vi "time_frequency.vi"() -> ()   [LabVIEW 2018]
uses:
  <vilib>/addons/Time Frequency Analysis/Spectrogram.llb/TFA Adaptive Spectrogram (Waveform).vi
  <vilib>/addons/Time Frequency Analysis/Spectrogram.llb/TFA Choi-Williams Distribution (Waveform).vi
  <vilib>/addons/Time Frequency Analysis/Transform.llb/TFA STFT (Waveform).vi
  <vilib>/addons/_Advanced Signal Processing/NI_AdvSigProcTFA.lvlib
  <vilib>/measure/NI_MABase.lvlib
panel:
  out "Waveform Graph 7":waveform(dbl)(graph)
  out "Waveform Graph 5":dbl[][](graph)
  out "Waveform Graph 4":dbl[][](graph)
  out "Waveform Graph 3":dbl[][](graph)
  in  "frequency":dbl=10.0 format="%0.2p"
  in  "window info":cluster{"type":i32, "length":i32}={"type"=1, "length"=-1} {"type" items=["None ", "Hanning", "Hamming", "Blackman-Harris", "Exact Blackman", "Blackman", "Flat Top", "4 Term B-Harris ", "7 Term B-Harris", "Low Sidelobe", "Gaussian"]}
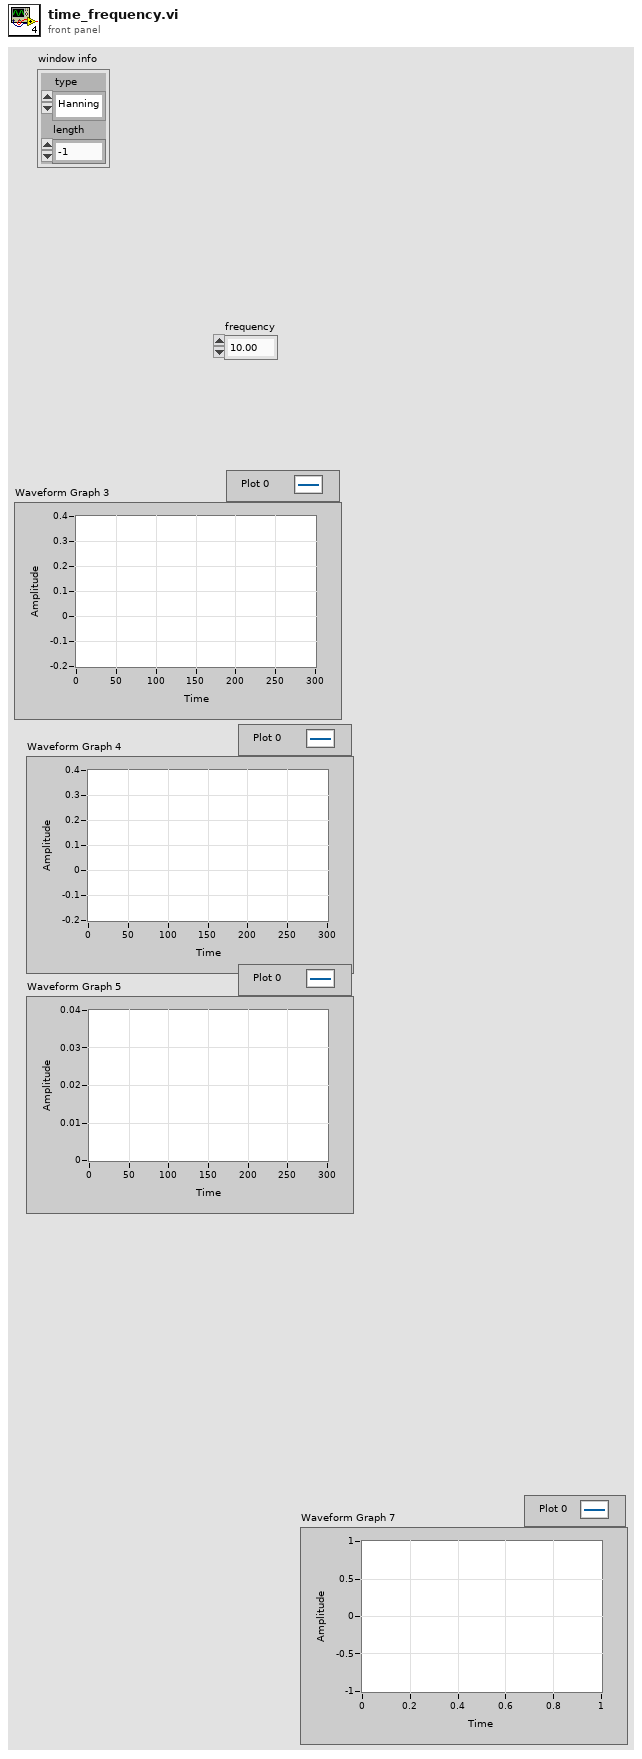
[diagram p1: front panel]
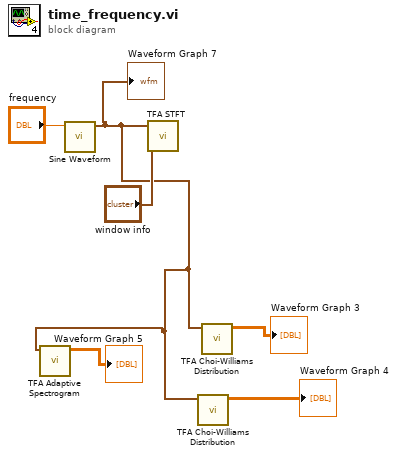
[diagram p0: block diagram]
diagram:
  n1 = call <vilib>:"Sine Waveform.vi"("frequency"="frequency") -> ("signal out"=w1:waveform(dbl))  [unwired: 9 in, 1 out]
  "Waveform Graph 7" <- w1
  n2 = call-poly <vilib>:"TFA Adaptive Spectrogram.vi"("signal"=w1) -> ("spectrogram"=→"Waveform Graph 5":dbl[][])  [unwired: 7 in, 3 out]
  n3 = call-poly <vilib>:"TFA STFT.vi"("window info"="window info", "signal"=w1) -> ()  [unwired: 7 in, 3 out]
  n4 = call-poly <vilib>:"TFA Choi-Williams Distribution.vi"("signal"=w1) -> ("spectrogram"=→"Waveform Graph 4":dbl[][])  [unwired: 8 in, 2 out]
  n5 = call-poly <vilib>:"TFA Choi-Williams Distribution.vi"("signal"=w1) -> ("spectrogram"=→"Waveform Graph 3":dbl[][])  [unwired: 8 in, 2 out]
